vi "Init.vi"(8 "error in (no error)":errorcluster, 11 "Scheduler in":refnum<class "Scheduler.lvclass">) -> (0 "error out":errorcluster, 3 "Scheduler out":refnum<class "Scheduler.lvclass">)   [LabVIEW 2020, in "Scheduler.lvlib" / "Scheduler.lvclass"]
uses:
  Scheduler.lvclass
  Scheduler Consumer Case Selector.ctl
  TALOS/TALOS_PPL.lvlibp/Support VIs/Global Memory.vi
  TALOS/TALOS_PPL.lvlibp/Father of all uServices/Father of all uServices/Father of all uServices.lvclass
  TALOS/TALOS_PPL.lvlibp
  C:/Users/aegis/Documents/CIRCUS/TALOS/TALOS_PPL.lvlibp/Father of all uServices/Father of all uServices/Father of all uServices.lvclass
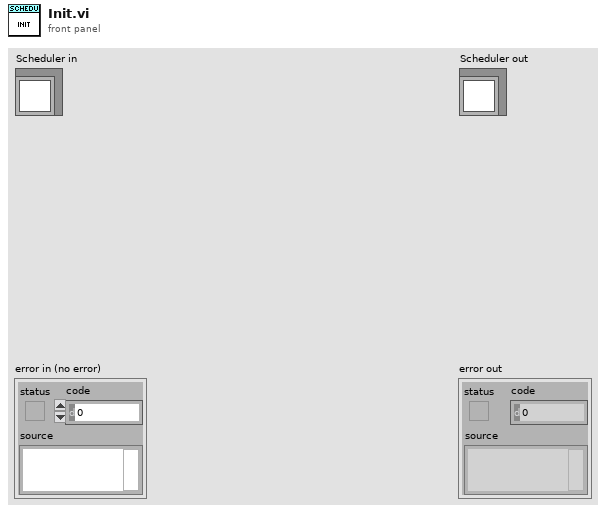
[diagram p1: front panel]
types:
  T1 = typedef "Scheduler.lvlib/Scheduler.lvclass/Scheduler Consumer Case Selector.ctl" = enum16{"Add SBlock", "Update GUI", "Move SBlock", "Select SBlock", "Update Cont.", "Load", "Save", "Reset", "Send to Tamer", "Edit SBlock", "Duplicate SBlock", "Delete SBlock", "Update SBlock", "Init", "Split/Combine Schedules", "Reschedule", "Load Parameters"}
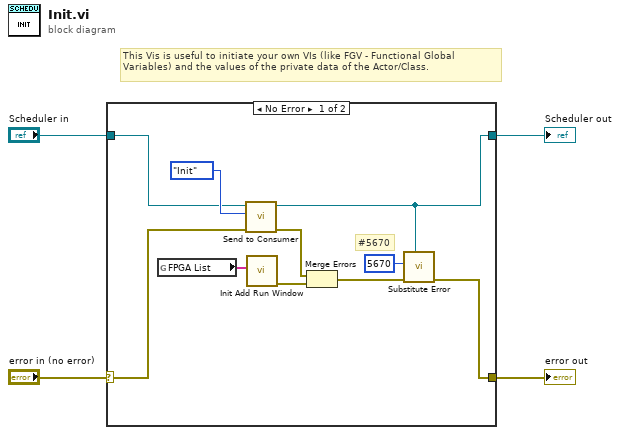
[diagram p0: block diagram]
diagram:
  # "This Vis is useful to initiate your own VIs (like FGV - Functional Global Variables) and the values of the private data of the Actor/Class."
  n1 = case shown="No Error" "error in (no error)" {
    selector: "error in (no error)" -> [w14 w15]
    tunnel: "Scheduler in" -> [w12 w16]
    tunnel: [w5 w16] -> w4
    tunnel: [w6 w15] -> w3
    frame No Error {
      # "#5670"
      n2 = global read "Global Memory.vi" "FPGA List"() -> (w10:string[])
      n3 = call "Send to Consumer.vi"("error in (no error)"=w14, "Case ID"=Scheduler_Consumer_Case_Selector."Init" ("Shifter Panel Consumer Case Selector"), "uService Template in"=w12) -> ("error out"=w8:errorcluster, "uService Template out"=w5:refnum<class "Scheduler.lvclass">)  [unwired: 7 in]
      n4 = call "Init Add Run Window.vi"("FPGA Names"=w10) -> ("error out"=w9:errorcluster)  [unwired: 10 in]
      n5 = Merge Errors(w8, w9) -> (w7:errorcluster)
      n6 = call "Substitute Error.vi"("LabVIEW Object"=w5, "error in (no error)"=w7, "Error Code"=5670) -> ("error out"=w6:errorcluster)  [unwired: 8 in]
    }
    frame Error {
    }
  }
  "error out" <- w3
  "Scheduler out" <- w4
